vi "Yokogawa wt 1600 device panel 4 Harmonic.vi"(2 "error in (no error)":errorcluster, 3 "Element":u16(ring)=1 items=["-", "Element 1", "Element 2", "Element 3", "Element 4", "Element 5", "Element 6", "Sigma A", "Sigma B", "Sigma C"], 4 "VISA session":refnum<visa-resource-name>) -> (0 "error out":errorcluster, 1 "dup VISA session":refnum<visa-resource-name>)   [LabVIEW 2012]
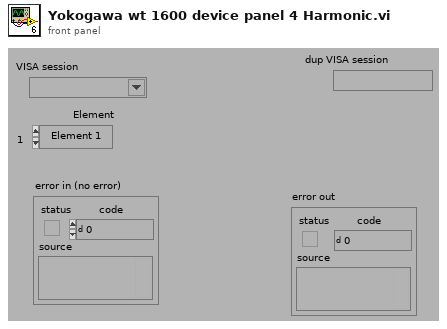
[diagram p1: front panel]
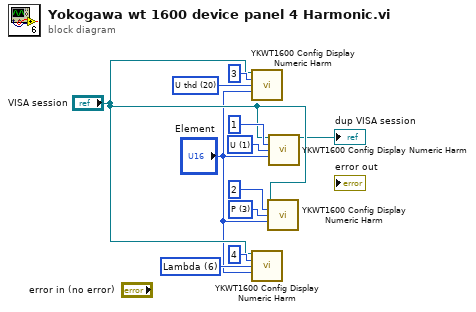
[diagram p0: block diagram]
diagram:
  w1 = u16 1 items=["None", "U", "I", "P", "S", "Q", "Lambda", "Phi", "Phi U", "Phi I", "Freq U", "Freq I", "Z", "Rs", "Xs", "Rp", "Xp", "U hdf", "I hdf", "P hdf", "U thd", "I thd", "P thd", "U thf", "I thf", "U thf", "I tif", "hvf", "hcf", "Phi U1-U2", "Phi U1-U3", "Phi U1-I1", "Phi U1-I2", "Phi U1-I3", "F1", "F2", "F3", "F4"] ("Display Function (0: None)")
  w3 = u16 6 items=["None", "U", "I", "P", "S", "Q", "Lambda", "Phi", "Phi U", "Phi I", "Freq U", "Freq I", "Z", "Rs", "Xs", "Rp", "Xp", "U hdf", "I hdf", "P hdf", "U thd", "I thd", "P thd", "U thf", "I thf", "U thf", "I tif", "hvf", "hcf", "Phi U1-U2", "Phi U1-U3", "Phi U1-I1", "Phi U1-I2", "Phi U1-I3", "F1", "F2", "F3", "F4"] ("Display Function (0: None)")
  w4 = u16 20 items=["None", "U", "I", "P", "S", "Q", "Lambda", "Phi", "Phi U", "Phi I", "Freq U", "Freq I", "Z", "Rs", "Xs", "Rp", "Xp", "U hdf", "I hdf", "P hdf", "U thd", "I thd", "P thd", "U thf", "I thf", "U thf", "I tif", "hvf", "hcf", "Phi U1-U2", "Phi U1-U3", "Phi U1-I1", "Phi U1-I2", "Phi U1-I3", "F1", "F2", "F3", "F4"] ("Display Function (0: None)")
  w5 = u16 3 items=["None", "U", "I", "P", "S", "Q", "Lambda", "Phi", "Phi U", "Phi I", "Freq U", "Freq I", "Z", "Rs", "Xs", "Rp", "Xp", "U hdf", "I hdf", "P hdf", "U thd", "I thd", "P thd", "U thf", "I thf", "U thf", "I tif", "hvf", "hcf", "Phi U1-U2", "Phi U1-U3", "Phi U1-I1", "Phi U1-I2", "Phi U1-I3", "F1", "F2", "F3", "F4"] ("Display Function (0: None)")
  n1 = call <instrlib>:"YKWT1600 Config Display Numeric Harm.vi"("VISA session"="VISA session", "Item Number (1)"=u16 3, "Display Function (0: None)"=w4, "Element (1: Element 1)"="Element") -> ()  [unwired: 10 in, 2 out]
  n2 = call <instrlib>:"YKWT1600 Config Display Numeric Harm.vi"("VISA session"="VISA session", "Item Number (1)"=u16 4, "Display Function (0: None)"=w3, "Element (1: Element 1)"="Element") -> ()  [unwired: 10 in, 2 out]
  n3 = call <instrlib>:"YKWT1600 Config Display Numeric Harm.vi"("VISA session"="VISA session", "Item Number (1)"=u16 2, "Display Function (0: None)"=w5, "Element (1: Element 1)"="Element") -> ()  [unwired: 10 in, 2 out]
  n4 = call <instrlib>:"YKWT1600 Config Display Numeric Harm.vi"("VISA session"="VISA session", "Item Number (1)"=u16 1, "Display Function (0: None)"=w1, "Element (1: Element 1)"="Element") -> ("dup VISA session"=→"dup VISA session":refnum<visa-resource-name>)  [unwired: 10 in, 1 out]
